vi "Begin.vi"(11 "Image Size":T1=enum."160x120") -> (0 "error out":errorcluster)   [LabVIEW 2012]
doc: "Called before other user functions, this VI is expected to open initial I/O refnums, load in file data, and do all program initialization. Notice that the <B>error out</B> terminal is simply used for data flow. Wiring it to other structures or subVIs ensures that this VI runs first."
uses:
  <vilib>/Rock Robotics/WPI/Camera/WPI_CameraImageSize.ctl
  <vilib>/Rock Robotics/WPI/Camera/WPI_CameraWhite Balance Values.ctl
  <vilib>/Rock Robotics/WPI/Camera/WPI_CameraExposure Values.ctl
  <vilib>/Rock Robotics/WPI/Camera/WPI_CameraFrameRate.ctl
  <vilib>/Rock Robotics/WPI/Joystick/WPI_JoystickDeviceEnum.ctl
  <vilib>/Rock Robotics/SystemInterfaces/DIO/FPGA_DIOPWMChannel.ctl
  <vilib>/Rock Robotics/SystemInterfaces/Typedef/FPGA_TypedefDigitalModule.ctl
  <vilib>/Rock Robotics/SystemInterfaces/DIO/FPGA_DIORelayChannel.ctl
  <vilib>/Rock Robotics/WPI/Relay/WPI_RelayDirection.ctl
  <vilib>/Rock Robotics/SystemInterfaces/AI/FPGA_AIGyroChannel.ctl
  <vilib>/Rock Robotics/SystemInterfaces/Typedef/FPGA_TypedefAnalogModuleForGyro.ctl
  <vilib>/Rock Robotics/WPI/AnalogChannel/WPI_AnalogChannelDevRef.ctl
  <vilib>/Rock Robotics/SystemInterfaces/Typedef/FPGA_TypedefAnalogModule.ctl
  <vilib>/Rock Robotics/SystemInterfaces/AI/FPGA_AIChannel.ctl
  <vilib>/Rock Robotics/SystemInterfaces/CounterEncoderSourceConvertion/FPGA_CounterEncoderSourceConvertionLVSourceType.ctl
  <vilib>/Rock Robotics/SystemInterfaces/DIO/FPGA_DIODigitalSourceChannel.ctl
  <vilib>/Rock Robotics/SystemInterfaces/AnalogTrigger/FPGA_AnalogTriggerIndex.ctl
  <vilib>/Rock Robotics/SystemInterfaces/AnalogTrigger/FPGA_AnalogTriggerOutType.ctl
  <vilib>/Rock Robotics/SystemInterfaces/DIO/FPGA_DIOChannel.ctl
  <vilib>/Rock Robotics/WPI/MotorControl/WPI_MotorControlOpen Jaguar.vi
  <vilib>/Rock Robotics/WPI/RobotDrive/WPI_RobotDriveOpen2MotorWithJaguar.vi
  <vilib>/Rock Robotics/WPI/MotorControl/WPI_MotorControlOpen Victor.vi
  <vilib>/Rock Robotics/WPI/Counter/WPI_CounterOpen UpDown Mode.vi
  <vilib>/Rock Robotics/WPI/Counter/WPI_CounterDigitalInputToDigitalSource.vi
  <vilib>/Rock Robotics/WPI/RobotDrive/WPI_RobotDriveOpen4MotorWithJaguar.vi
panel:
  out "error out 2":errorcluster
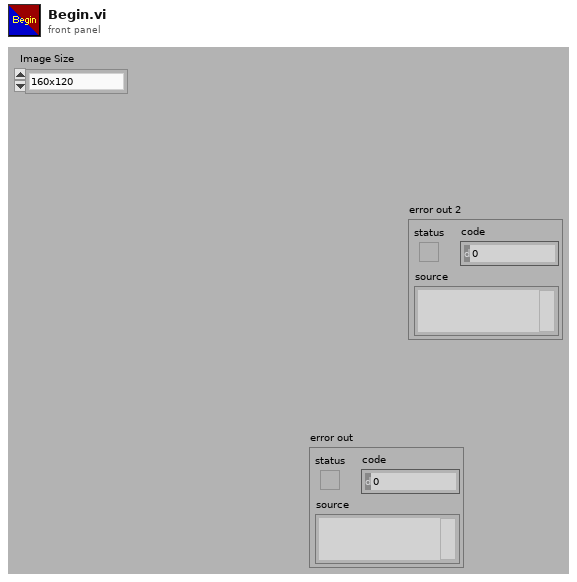
[diagram p1: front panel]
types:
  T1 = typedef "WPI_CameraImageSize.ctl" = enum16{"640x480", "320x240", "160x120"}
  T2 = typedef "FPGA_DIOPWMChannel.ctl" = enum8{"PWM 1", "PWM 2", "PWM 3", "PWM 4", "PWM 5", "PWM 6", "PWM 7", "PWM 8", "PWM 9", "PWM 10", "Invalid"}
  T3 = typedef "FPGA_TypedefDigitalModule.ctl" = enum16{"Digital Module 1", "Digital Module 2"}
  T4 = typedef "WPI_RelayDirection.ctl" = enum16{"Both directions", "Forward only", "Reverse only"}
  T5 = typedef "FPGA_DIORelayChannel.ctl" = enum8{"Relay 1", "Relay 2", "Relay 3", "Relay 4", "Relay 5", "Relay 6", "Relay 7", "Relay 8", "Invalid"}
  T6 = typedef "WPI_JoystickDeviceEnum.ctl" = enum16{"USB 1", "USB 2", "USB 3", "USB 4", "Kinect 1", "Kinect 2"}
  T7 = typedef "WPI_CameraFrameRate.ctl" = u32
  T8 = typedef "WPI_CameraExposure Values.ctl" = enum16{"Auto", "Flicker-free 50 Hz", "Flicker-free 60 Hz", "Hold current"}
  T9 = typedef "WPI_CameraWhite Balance Values.ctl" = enum16{"Auto", "Fixed indoor", "Fixed outdoor 1", "Fixed outdoor 2", "Fixed fluorescent 1", "Fixed fluorescent 2", "Hold current"}
  T10 = typedef "WPI_ServoDeviceRef.ctl" = cluster{"DeviceStatus":errorcluster, "Digital Module":T3, "PWM Channel":T2, "DeadBand":T11}
  T11 = typedef "WPI_PWMDeadband.ctl" = cluster{"Name":string, "maxPositivePwm":i32, "minPositivePwm":i32, "centerPwm":i32, "maxNegativePwm":i32, "minNegativePwm":i32, "angularRange":u16}
  T12 = typedef "WPI_MotorControlDeviceRef.ctl" = cluster{"DeviceStatus":errorcluster, "Type":enum16{"PWM", "CAN"}, "PWM":cluster{"Digital Module":T3, "PWM Channel":T2, "DeadBand":T11}, "CAN":cluster{"Device Number":u8, "Control Mode":T13, "Semaphore":T14, "Max Vout":dbl}, "Invert":bool, "TransformRef":T15, "InvTransformRef":T15}
  T13 = typedef "WPI_CANJaguar_ControlMode.ctl" = enum8{"Percent VBus", "Current", "Speed", "Position", "Voltage"}
  T14 = typedef "Semaphore RefNum" = refnum<k1>
  T15 = typedef "WPI_PWMTransform_ConPane.ctl" = refnum<vi>
  T16 = enum16{"Rising Edge", "Falling Edge", "Raising & Falling Edge", "Disabled"}
  T17 = typedef "FPGA_CounterEncoderSourceConvertionLVSourceType.ctl" = cluster{"DevStatus":errorcluster, "AnalogTriggerMode?":bool, "DigitalMode":cluster{"Digital Module":T3, "DIO Channel":T18}, "AnalogTriggerMode":cluster{"AnalogTriggerIndex":T19, "OutputType":T20}}
  T18 = typedef "FPGA_DIODigitalSourceChannel.ctl" = enum8{"DIO 1", "DIO 2", "DIO 3", "DIO 4", "DIO 5", "DIO 6", "DIO 7", "DIO 8", "DIO 9", "DIO 10", "DIO 11", "DIO 12", "DIO 13", "DIO 14", "Disabled"}
  T19 = typedef "FPGA_AnalogTriggerIndex.ctl" = enum8{"Trig 0", "Trig 1", "Trig 2", "Trig 3", "Trig 4", "Trig 5", "Trig 6", "Trig 7", "Invalid"}
  T20 = typedef "FPGA_AnalogTriggerOutType.ctl" = enum16{"InWindow", "TriggerState", "Rising", "Falling"}
  T21 = typedef "WPI_AnalogChannelDevRef.ctl" = cluster{"DevStatus":errorcluster, "Analog Module":T22, "Analog Channel":T23}
  T22 = typedef "FPGA_TypedefAnalogModule.ctl" = enum16{"Analog Module 1", "Analog Module 2"}
  T23 = typedef "FPGA_AIChannel.ctl" = enum8{"AI 1", "AI 2", "AI 3", "AI 4", "AI 5", "AI 6", "AI 7", "AI 8", "Invalid"}
  T24 = typedef "FPGA_AnalogTriggerDevRef.ctl" = cluster{"DevStatus":errorcluster, "AnalogTriggerIndex":T19}
  T25 = typedef "WPI_CounterDevRef.ctl" = cluster{"DevStatus":errorcluster, "CntIndex":T26}
  T26 = typedef "FPGA_CounterCtrSystemIndex.ctl" = enum8{"Ctr 0", "Ctr 1", "Ctr 2", "Ctr 3", "Ctr 4", "Ctr 5", "Ctr 6", "Ctr 7", "Invalid"}
  T27 = typedef "WPI_RobotDriveDevRef.ctl" = cluster{"DevStatus":errorcluster, "Motors[]":T12[], "Square Inputs":bool, "Max Output":dbl, "Isochronous":bool}
  T28 = typedef "FPGA_DIOChannel.ctl" = enum8{"DIO 1", "DIO 2", "DIO 3", "DIO 4", "DIO 5", "DIO 6", "DIO 7", "DIO 8", "DIO 9", "DIO 10", "DIO 11", "DIO 12", "DIO 13", "DIO 14", "Invalid"}
  T29 = typedef "WPI_DigitalInputDevRef.ctl" = cluster{"DevStatus":errorcluster, "DIO Channel":T28, "Digital Module":T3}
  T30 = typedef "WPI_CameraDevRef.ctl" = cluster{"Camera Address":string, "CameraStatus":errorcluster, "Acquire Image Notifier":refnum<notifier>}
  T31 = typedef "WPI_JoystickDevRef.ctl" = cluster{"Device":T6}
  T32 = typedef "WPI_RelayDevRef.ctl" = cluster{"DevStatus":errorcluster, "Relay Channel":T5, "Digital Module":T3, "Relay Direction":T4}
  T33 = typedef "FPGA_AIGyroChannel.ctl" = enum8{"AI 1", "AI 2", "Invalid"}
  T34 = typedef "FPGA_TypedefAnalogModuleForGyro.ctl" = enum16{"Analog Module 1"}
  T35 = typedef "WPI_GyroDevRef.ctl" = cluster{"DevStatus":errorcluster, "Analog Module":T22, "Analog Channel":T23, "Offset":dbl, "Gain (VoltsPerDegree/Second)":dbl}
  T36 = typedef "WPI_EncoderDevRef.ctl" = cluster{"DevStatus":errorcluster, "EncoderIndex":T37, "CounterIndex":T26, "DistancePerCount":dbl, "Decoding Type":T38}
  T37 = typedef "FPGA_EncoderIdx.ctl" = enum8{"Enc 0", "Enc 1", "Enc 2", "Enc 3", "Invalid"}
  T38 = typedef "WPI_EncoderType.ctl" = enum16{"1x", "2x", "4x"}
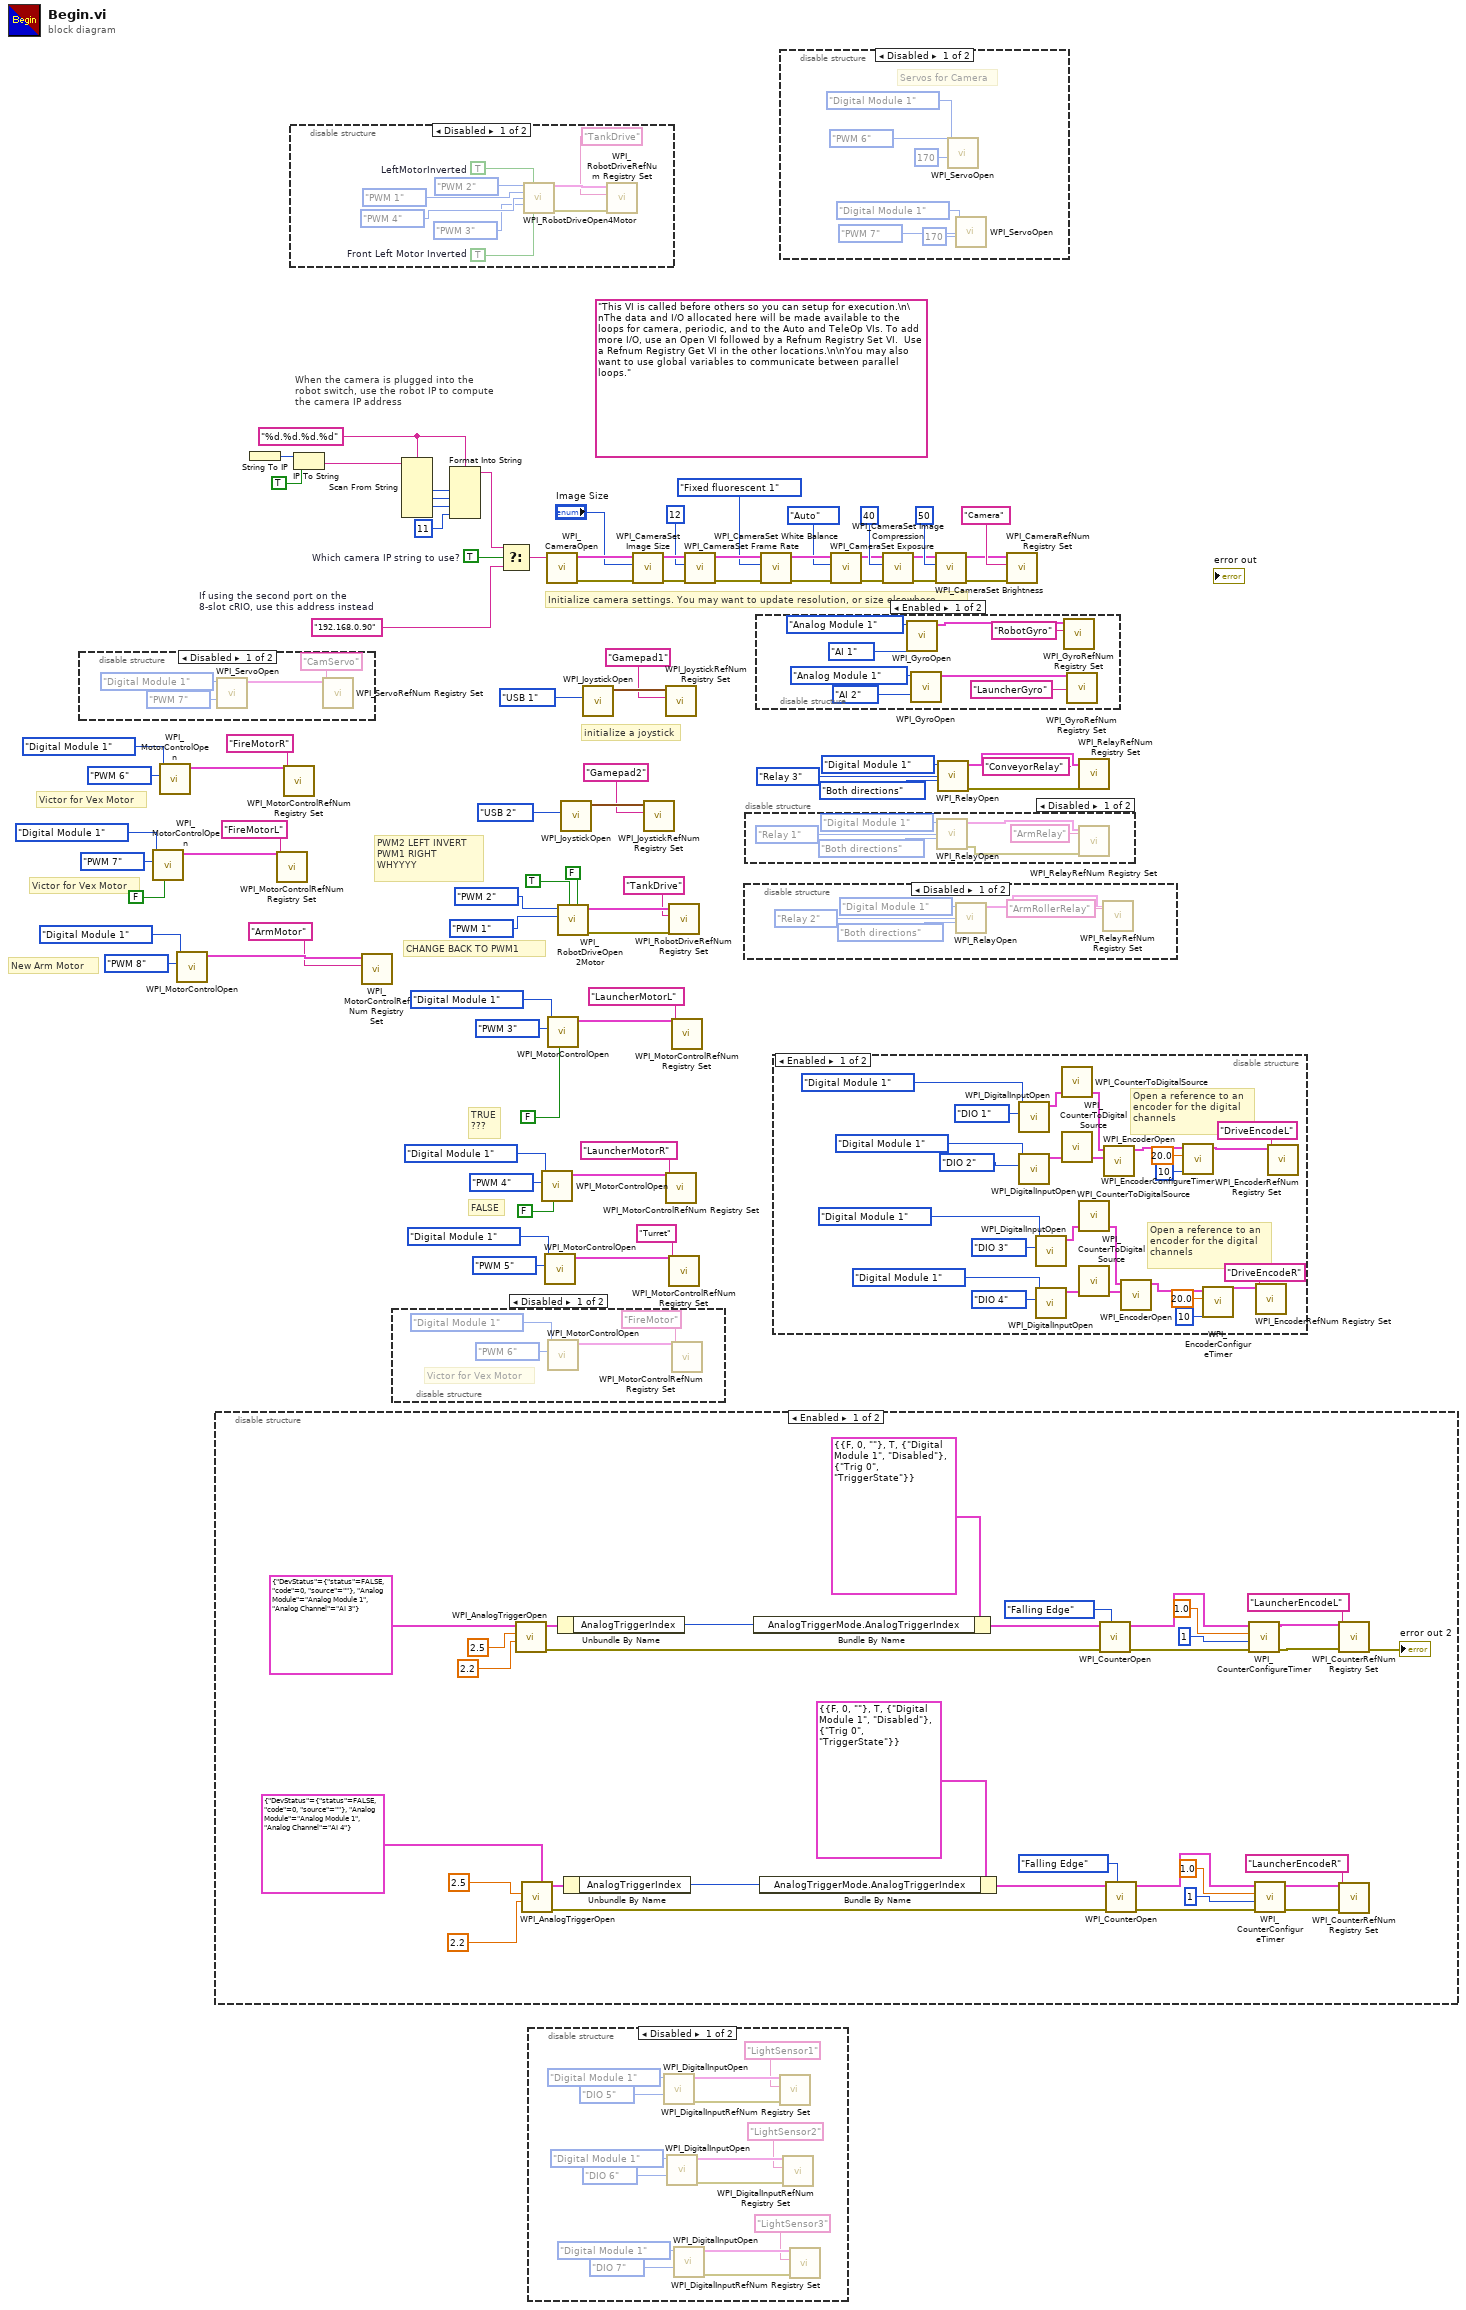
[diagram p0: block diagram]
diagram:
  w47 = TRUE  # Which camera IP string to use?
  w51 = "%d.%d.%d.%d" ("format string")
  (unwired) "This VI is called before others so you can setup for execution.\n\nThe data and I/O allocated here will be made available to the loops for camera, periodic, and to the Auto and TeleOp VIs. To add more I/O, use an Open VI followed by a Refnum Registry Set VI.  Use a Refnum Registry Get VI in the other locations.\n\nYou may also want to use global variables to communicate between parallel loops."
  w48 = "192.168.0.90"  # If using the second port on the 8-slot cRIO, use this address instead
  # "New Arm Motor"
  # "Victor for Vex Motor"
  # "Victor for Vex Motor"
  # "FALSE"
  # "TRUE\n???"
  # "PWM2 LEFT INVERT\nPWM1 RIGHT\nWHYYYY"
  # "CHANGE BACK TO PWM1"
  # "initialize a joystick"
  # "When the camera is plugged into the\nrobot switch, use the robot IP to compute\nthe camera IP address"
  # "Initialize camera settings. You may want to update resolution, or size elsewhere."
  n1 = disable-structure shown="Disabled" {
    frame Disabled {
      n2 = call <vilib>:"WPI_ServoOpen.vi"("PWM Channel"=FPGA_DIOPWMChannel."PWM 7", "Digital Module (Module 1)"=FPGA_TypedefDigitalModule."Digital Module 1") -> ("ServoDeviceRef"=w83:T10)  [unwired: 8 in, 1 out]
      n3 = call <vilib>:"WPI_ServoRefNum Registry Set.vi"("refnum name"="CamServo", "ServoDeviceRef"=w83) -> ()  [unwired: 8 in, 2 out]
    }
    frame Enabled {
    }
  }
  n4 = call-poly <vilib>:"WPI_MotorControlOpen.vi"("Invert"=FALSE, "PWM Channel"=FPGA_DIOPWMChannel."PWM 7", "Digital Module (Module 1)"=FPGA_TypedefDigitalModule."Digital Module 1") -> ("MotorControlDeviceRef"=w7:T12)  [unwired: 7 in, 1 out]
  n5 = call-poly <vilib>:"WPI_MotorControlOpen.vi"("PWM Channel"=FPGA_DIOPWMChannel."PWM 6", "Digital Module (Module 1)"=FPGA_TypedefDigitalModule."Digital Module 1") -> ("MotorControlDeviceRef"=w11:T12)  [unwired: 8 in, 1 out]
  n6 = call-poly <vilib>:"WPI_MotorControlOpen.vi"("PWM Channel"=FPGA_DIOPWMChannel."PWM 8", "Digital Module (Module 1)"=FPGA_TypedefDigitalModule."Digital Module 1") -> ("MotorControlDeviceRef"=w2:T12)  [unwired: 8 in, 1 out]
  n7 = disable-structure shown="Enabled" {
    frame Enabled {
      n8 = call <vilib>:"WPI_AnalogTriggerOpen.vi"("LowerLimit (v)"=2.2, "UpperLimit (v)"=2.5, "AnalogTriggerSource"=T21 {"DevStatus"={"status"=FALSE, "code"=0, "source"=""}, "Analog Module"=enum."Analog Module 1", "Analog Channel"=enum."AI 3"}) -> ("error out"=w115:errorcluster, "AnalogTriggerDevRef"=w108:T24)  [unwired: 7 in]
      n9 = call <vilib>:"WPI_AnalogTriggerOpen.vi"("LowerLimit (v)"=2.2 ("LowerLimit (v) 2"), "UpperLimit (v)"=2.5 ("UpperLimit (v) 2"), "AnalogTriggerSource"=T21 {"DevStatus"={"status"=FALSE, "code"=0, "source"=""}, "Analog Module"=enum."Analog Module 1", "Analog Channel"=enum."AI 4"} ("AnalogTriggerSource 2")) -> ("error out"=w102:errorcluster, "AnalogTriggerDevRef"=w95:T24)  [unwired: 7 in]
      n10 = Unbundle By Name(w108) -> ("AnalogTriggerIndex"=w107:T19)
      n11 = Unbundle By Name(w95) -> ("AnalogTriggerIndex"=w94:T19)
      n12 = Bundle By Name(cluster=T17 {"DevStatus"={"status"=FALSE, "code"=0, "source"=""}, "AnalogTriggerMode?"=TRUE, "DigitalMode"={"Digital Module"=enum."Digital Module 1", "DIO Channel"=enum."Disabled"}, "AnalogTriggerMode"={"AnalogTriggerIndex"=enum."Trig 0", "OutputType"=enum."TriggerState"}} ("Source"), "AnalogTriggerMode.AnalogTriggerIndex"=w107) -> (w105:T17)
      n13 = Bundle By Name(cluster=T17 {"DevStatus"={"status"=FALSE, "code"=0, "source"=""}, "AnalogTriggerMode?"=TRUE, "DigitalMode"={"Digital Module"=enum."Digital Module 1", "DIO Channel"=enum."Disabled"}, "AnalogTriggerMode"={"AnalogTriggerIndex"=enum."Trig 0", "OutputType"=enum."TriggerState"}} ("Source 2"), "AnalogTriggerMode.AnalogTriggerIndex"=w94) -> (w92:T17)
      n14 = call-poly <vilib>:"WPI_CounterOpen.vi"("UpEdge"=T16."Falling Edge" ("UpEdge 1"), "error in (no error)"=w115, "Up Source"=w105) -> ("error out"=w111:errorcluster, "CounterDevRef"=w112:T25)  [unwired: 7 in]
      n15 = call-poly <vilib>:"WPI_CounterOpen.vi"("UpEdge"=T16."Falling Edge" ("UpEdge 2"), "error in (no error)"=w102, "Up Source"=w92) -> ("error out"=w98:errorcluster, "CounterDevRef"=w99:T25)  [unwired: 7 in]
      n16 = call <vilib>:"WPI_CounterConfigureTimer.vi"("error in (no error)"=w111, "Number Samples to Average"=u8 1, "MaxPeriod (sec)"=1.0, "CounterDevRef in"=w112) -> ("error out"=w85:errorcluster, "CounterDevRef out"=w86:T25)  [unwired: 6 in]
      n17 = call <vilib>:"WPI_CounterConfigureTimer.vi"("error in (no error)"=w98, "Number Samples to Average"=u8 1, "MaxPeriod (sec)"=1.0, "CounterDevRef in"=w99) -> ("error out"=w89:errorcluster, "CounterDevRef out"=w90:T25)  [unwired: 6 in]
      n18 = call <vilib>:"WPI_CounterRefNum Registry Set.vi"("error in (no error)"=w85, "refnum name"="LauncherEncodeL", "CounterDevRef"=w86) -> ("error out"=→"error out 2":errorcluster)  [unwired: 7 in, 1 out]
      n19 = call <vilib>:"WPI_CounterRefNum Registry Set.vi"("error in (no error)"=w89, "refnum name"="LauncherEncodeR", "CounterDevRef"=w90) -> ()  [unwired: 7 in, 2 out]
    }
    frame Disabled {
    }
  }
  n20 = String To IP() -> (0:w58:u32)  [unwired: 1 in]
  n21 = call <vilib>:"WPI_MotorControlRefNum Registry Set.vi"("refnum name"="FireMotorL", "MotorControlDevRef"=w7) -> ()  [unwired: 8 in, 2 out]
  n22 = call <vilib>:"WPI_MotorControlRefNum Registry Set.vi"("refnum name"="FireMotorR", "MotorControlDevRef"=w11) -> ()  [unwired: 8 in, 2 out]
  n23 = disable-structure shown="Disabled" {
    frame Disabled {
      w119 = TRUE  # Front Left Motor Inverted
      w125 = TRUE  # LeftMotorInverted
      n24 = call-poly <vilib>:"WPI_RobotDriveOpen4Motor.vi"("Rear Left Motor"=FPGA_DIOPWMChannel."PWM 2" ("Left"), "Rear Left Motor Inverted"=w125, "Rear Right Motor"=FPGA_DIOPWMChannel."PWM 1" ("Right Motor"), "Front Left Motor"=FPGA_DIOPWMChannel."PWM 4", "Front Right Motor"=FPGA_DIOPWMChannel."PWM 3", "Front Left Motor Inverted"=w119) -> ("RobotDriveDevRef"=w124:T27, "error out"=w122:errorcluster)  [unwired: 8 in]
      n25 = call <vilib>:"WPI_RobotDriveRefNum Registry Set.vi"("error in (no error)"=w122, "refnum name"="TankDrive", "RobotDriveDevRef"=w124) -> ()  [unwired: 9 out]
    }
    frame Enabled {
    }
  }
  n26 = IP To String(1:TRUE ("dot notation? (F)"), 2:w58) -> (0:w56:string)
  n27 = call <vilib>:"WPI_MotorControlRefNum Registry Set.vi"("refnum name"="ArmMotor", "MotorControlDevRef"=w2) -> ()  [unwired: 8 in, 2 out]
  n28 = disable-structure shown="Disabled" {
    frame Disabled {
      # "Victor for Vex Motor"
      n29 = call-poly <vilib>:"WPI_MotorControlOpen.vi"("PWM Channel"=FPGA_DIOPWMChannel."PWM 6", "Digital Module (Module 1)"=FPGA_TypedefDigitalModule."Digital Module 1") -> ("MotorControlDeviceRef"=w127:T12)  [unwired: 8 in, 1 out]
      n30 = call <vilib>:"WPI_MotorControlRefNum Registry Set.vi"("refnum name"="FireMotor", "MotorControlDevRef"=w127) -> ()  [unwired: 8 in, 2 out]
    }
    frame Enabled {
    }
  }
  n31 = Scan From String(format string=w51, input string=w56) -> (output 1=w55:i32, output 2=w54:i32, output 3=w53:i32)  [unwired: 7 in, 3 out]
  n32 = Format Into String(format string=w51, w55, w54, w53, 11 ("Compression")) -> (resulting string=w49:string)  [unwired: 2 in, 1 out]
  n33 = Select(t=w49, s=w47, f=w48) -> (s? t:f=w50:string)
  n34 = disable-structure shown="Disabled" {
    frame Disabled {
      n35 = call <vilib>:"WPI_DigitalInputOpen.vi"("DIO Channel"=FPGA_DIOChannel."DIO 5", "Digital Module (Module 1)"=FPGA_TypedefDigitalModule."Digital Module 1") -> ("error out"=w141:errorcluster, "DigitalInputDevRef"=w142:T29)  [unwired: 8 in]
      n36 = call <vilib>:"WPI_DigitalInputOpen.vi"("DIO Channel"=FPGA_DIOChannel."DIO 6", "Digital Module (Module 1)"=FPGA_TypedefDigitalModule."Digital Module 1") -> ("error out"=w136:errorcluster, "DigitalInputDevRef"=w137:T29)  [unwired: 8 in]
      n37 = call <vilib>:"WPI_DigitalInputOpen.vi"("DIO Channel"=FPGA_DIOChannel."DIO 7", "Digital Module (Module 1)"=FPGA_TypedefDigitalModule."Digital Module 1") -> ("error out"=w131:errorcluster, "DigitalInputDevRef"=w132:T29)  [unwired: 8 in]
      n38 = call <vilib>:"WPI_DigitalInputRefNum Registry Set.vi"("error in (no error)"=w141, "refnum name"="LightSensor1", "DigitalInputDevRef"=w142) -> ()  [unwired: 7 in, 2 out]
      n39 = call <vilib>:"WPI_DigitalInputRefNum Registry Set.vi"("error in (no error)"=w136, "refnum name"="LightSensor2", "DigitalInputDevRef"=w137) -> ()  [unwired: 7 in, 2 out]
      n40 = call <vilib>:"WPI_DigitalInputRefNum Registry Set.vi"("error in (no error)"=w131, "refnum name"="LightSensor3", "DigitalInputDevRef"=w132) -> ()  [unwired: 7 in, 2 out]
    }
    frame Enabled {
    }
  }
  n41 = call-poly <vilib>:"WPI_MotorControlOpen.vi"("Invert"=FALSE, "PWM Channel"=FPGA_DIOPWMChannel."PWM 4", "Digital Module (Module 1)"=FPGA_TypedefDigitalModule."Digital Module 1") -> ("MotorControlDeviceRef"=w29:T12)  [unwired: 7 in, 1 out]
  n42 = call-poly <vilib>:"WPI_MotorControlOpen.vi"("PWM Channel"=FPGA_DIOPWMChannel."PWM 5", "Digital Module (Module 1)"=FPGA_TypedefDigitalModule."Digital Module 1") -> ("MotorControlDeviceRef"=w25:T12)  [unwired: 8 in, 1 out]
  n43 = call <vilib>:"WPI_CameraOpen.vi"("Camera Address"=w50) -> ("error out"=w70:errorcluster, "CameraDevRef"=w71:T30)  [unwired: 1 in, 8 out]
  n44 = call-poly <vilib>:"WPI_MotorControlOpen.vi"("Invert"=FALSE, "PWM Channel"=FPGA_DIOPWMChannel."PWM 3", "Digital Module (Module 1)"=FPGA_TypedefDigitalModule."Digital Module 1") -> ("MotorControlDeviceRef"=w33:T12)  [unwired: 7 in, 1 out]
  n45 = call-poly <vilib>:"WPI_RobotDriveOpen2Motor.vi"("Right Motor Inverted"=FALSE, "Left Motor Inverted"=TRUE, "Right Motor"=FPGA_DIOPWMChannel."PWM 1", "Left Motor"=FPGA_DIOPWMChannel."PWM 2") -> ("error out"=w36:errorcluster, "RobotDriveDevRef"=w40:T27)  [unwired: 6 in]
  n46 = call <vilib>:"WPI_JoystickOpen.vi"("JoystickDevice"=WPI_JoystickDeviceEnum."USB 2") -> ("JoystickDevRef"=w43:T31)  [unwired: 10 out]
  n47 = call <vilib>:"WPI_JoystickOpen.vi"("JoystickDevice"=WPI_JoystickDeviceEnum."USB 1") -> ("JoystickDevRef"=w46:T31)  [unwired: 10 out]
  n48 = call <vilib>:"WPI_CameraSet Image Size.vi"("error in (no error)"=w70, "Image Size"="Image Size", "CameraDevRef"=w71) -> ("error out"=w69:errorcluster, "CameraDevRef Out"=w72:T30)  [unwired: 7 out]
  n49 = call <vilib>:"WPI_JoystickRefNum Registry Set.vi"("refnum name"="Gamepad2", "JoystickDevRef"=w43) -> ()  [unwired: 1 in, 9 out]
  n50 = call <vilib>:"WPI_JoystickRefNum Registry Set.vi"("refnum name"="Gamepad1", "JoystickDevRef"=w46) -> ()  [unwired: 1 in, 9 out]
  n51 = call <vilib>:"WPI_MotorControlRefNum Registry Set.vi"("refnum name"="LauncherMotorR", "MotorControlDevRef"=w29) -> ()  [unwired: 8 in, 2 out]
  n52 = call <vilib>:"WPI_RobotDriveRefNum Registry Set.vi"("error in (no error)"=w36, "refnum name"="TankDrive", "RobotDriveDevRef"=w40) -> ()  [unwired: 7 in, 2 out]
  n53 = call <vilib>:"WPI_MotorControlRefNum Registry Set.vi"("refnum name"="Turret", "MotorControlDevRef"=w25) -> ()  [unwired: 8 in, 2 out]
  n54 = call <vilib>:"WPI_MotorControlRefNum Registry Set.vi"("refnum name"="LauncherMotorL", "MotorControlDevRef"=w33) -> ()  [unwired: 8 in, 2 out]
  n55 = call <vilib>:"WPI_CameraSet Frame Rate.vi"("error in (no error)"=w69, "Frame Rate (fps)"=T7 12, "CameraDevRef"=w72) -> ("error out"=w68:errorcluster, "CameraDevRef Out"=w74:T30)  [unwired: 7 out]
  n56 = disable-structure shown="Disabled" {
    frame Disabled {
      n57 = call <vilib>:"WPI_RelayOpen.vi"("Relay Direction"=WPI_RelayDirection."Both directions", "Relay Channel"=FPGA_DIORelayChannel."Relay 2", "Digital Module (Module 1)"=FPGA_TypedefDigitalModule."Digital Module 1") -> ("RelayDevRef"=w145:T32)  [unwired: 7 in, 1 out]
      n58 = call <vilib>:"WPI_RelayRefNum Registry Set.vi"("refnum name"="ArmRollerRelay", "RelayDevRef"=w145) -> ()  [unwired: 8 in, 2 out]
    }
    frame Enabled {
    }
  }
  n59 = disable-structure shown="Disabled" {
    frame Disabled {
      n60 = call <vilib>:"WPI_RelayOpen.vi"("Relay Direction"=WPI_RelayDirection."Both directions", "Relay Channel"=FPGA_DIORelayChannel."Relay 1", "Digital Module (Module 1)"=FPGA_TypedefDigitalModule."Digital Module 1") -> ("error out"=w150:errorcluster, "RelayDevRef"=w151:T32)  [unwired: 7 in]
      n61 = call <vilib>:"WPI_RelayRefNum Registry Set.vi"("error in (no error)"=w150, "refnum name"="ArmRelay", "RelayDevRef"=w151) -> ()  [unwired: 7 in, 2 out]
    }
    frame Enabled {
    }
  }
  n62 = disable-structure shown="Enabled" {
    frame Enabled {
      n63 = call <vilib>:"WPI_GyroOpen.vi"("Analog Channel"=FPGA_AIGyroChannel."AI 1", "Analog Module (Module 1)"=FPGA_TypedefAnalogModuleForGyro."Analog Module 1") -> ("GyroDevRef"=w159:T35)  [unwired: 7 in, 2 out]
      n64 = call <vilib>:"WPI_GyroOpen.vi"("Analog Channel"=FPGA_AIGyroChannel."AI 2", "Analog Module (Module 1)"=FPGA_TypedefAnalogModuleForGyro."Analog Module 1") -> ("GyroDevRef"=w158:T35)  [unwired: 7 in, 2 out]
      n65 = call <vilib>:"WPI_GyroRefNum Registry Set.vi"("refnum name"="RobotGyro", "GyroDevRef"=w159) -> ()  [unwired: 8 in, 2 out]
      n66 = call <vilib>:"WPI_GyroRefNum Registry Set.vi"("refnum name"="LauncherGyro", "GyroDevRef"=w158) -> ()  [unwired: 8 in, 2 out]
    }
    frame Disabled {
    }
  }
  n67 = call <vilib>:"WPI_CameraSet White Balance.vi"("error in (no error)"=w68, "White Balance"=WPI_CameraWhite_Balance_Values."Fixed fluorescent 1", "CameraDevRef"=w74) -> ("error out"=w67:errorcluster, "CameraDevRef Out"=w73:T30)  [unwired: 7 out]
  n68 = disable-structure shown="Enabled" {
    frame Enabled {
      # "Open a reference to an\nencoder for the digital \nchannels"
      # "Open a reference to an\nencoder for the digital \nchannels"
      n69 = call <vilib>:"WPI_DigitalInputOpen.vi"("DIO Channel"=FPGA_DIOChannel."DIO 1", "Digital Module (Module 1)"=FPGA_TypedefDigitalModule."Digital Module 1") -> ("DigitalInputDevRef"=w187:T29)  [unwired: 1 in, 8 out]
      n70 = call <vilib>:"WPI_DigitalInputOpen.vi"("DIO Channel"=FPGA_DIOChannel."DIO 2", "Digital Module (Module 1)"=FPGA_TypedefDigitalModule."Digital Module 1") -> ("DigitalInputDevRef"=w188:T29)  [unwired: 1 in, 8 out]
      n71 = call <vilib>:"WPI_DigitalInputOpen.vi"("DIO Channel"=FPGA_DIOChannel."DIO 3", "Digital Module (Module 1)"=FPGA_TypedefDigitalModule."Digital Module 1") -> ("DigitalInputDevRef"=w177:T29)  [unwired: 1 in, 8 out]
      n72 = call <vilib>:"WPI_DigitalInputOpen.vi"("DIO Channel"=FPGA_DIOChannel."DIO 4", "Digital Module (Module 1)"=FPGA_TypedefDigitalModule."Digital Module 1") -> ("DigitalInputDevRef"=w178:T29)  [unwired: 1 in, 8 out]
      n73 = call-poly <vilib>:"WPI_CounterToDigitalSource.vi"("DigitalInputDevRef"=w187) -> ("Digital Source"=w186:T17)  [unwired: 6 out]
      n74 = call-poly <vilib>:"WPI_CounterToDigitalSource.vi"("DigitalInputDevRef"=w188) -> ("Digital Source"=w189:T17)  [unwired: 6 out]
      n75 = call-poly <vilib>:"WPI_CounterToDigitalSource.vi"("DigitalInputDevRef"=w177) -> ("Digital Source"=w176:T17)  [unwired: 6 out]
      n76 = call-poly <vilib>:"WPI_CounterToDigitalSource.vi"("DigitalInputDevRef"=w178) -> ("Digital Source"=w179:T17)  [unwired: 6 out]
      n77 = call <vilib>:"WPI_EncoderOpen.vi"("BSource"=w189, "ASource"=w186) -> ("EncoderDevRef"=w183:T36)  [unwired: 6 in, 3 out]
      n78 = call <vilib>:"WPI_EncoderOpen.vi"("BSource"=w179, "ASource"=w176) -> ("EncoderDevRef"=w175:T36)  [unwired: 6 in, 3 out]
      n79 = call <vilib>:"WPI_EncoderConfigureTimer.vi"("Number Samples to Average"=u8 10, "Minimum Rate"=20.0, "EncoderDevRef"=w183) -> ("EncoderDevRef"=w180:T36)  [unwired: 1 in, 7 out]
      n80 = call <vilib>:"WPI_EncoderConfigureTimer.vi"("Number Samples to Average"=u8 10, "Minimum Rate"=20.0, "EncoderDevRef"=w175) -> ("EncoderDevRef"=w172:T36)  [unwired: 1 in, 7 out]
      n81 = call <vilib>:"WPI_EncoderRefNum Registry Set.vi"("refnum name"="DriveEncodeR", "EncoderDevRef"=w172) -> ()  [unwired: 8 in, 2 out]
      n82 = call <vilib>:"WPI_EncoderRefNum Registry Set.vi"("refnum name"="DriveEncodeL", "EncoderDevRef"=w180) -> ()  [unwired: 8 in, 2 out]
    }
    frame Disabled {
    }
  }
  n83 = disable-structure shown="Disabled" {
    frame Disabled {
      # "Servos for Camera"
      n84 = call <vilib>:"WPI_ServoOpen.vi"("Angular Range"=u16 170, "PWM Channel"=FPGA_DIOPWMChannel."PWM 6", "Digital Module (Module 1)"=FPGA_TypedefDigitalModule."Digital Module 1") -> ()  [unwired: 7 in, 2 out]
      n85 = call <vilib>:"WPI_ServoOpen.vi"("Angular Range"=u16 170, "PWM Channel"=FPGA_DIOPWMChannel."PWM 7", "Digital Module (Module 1)"=FPGA_TypedefDigitalModule."Digital Module 1") -> ()  [unwired: 7 in, 2 out]
    }
    frame Enabled {
    }
  }
  n86 = call <vilib>:"WPI_CameraSet Exposure.vi"("error in (no error)"=w67, "Exposure"=WPI_CameraExposure_Values."Auto", "CameraDevRef"=w73) -> ("error out"=w66:errorcluster, "CameraDevRef Out"=w76:T30)  [unwired: 7 out]
  n87 = call <vilib>:"WPI_CameraSet Image Compression.vi"("error in (no error)"=w66, "Compression"=40, "CameraDevRef"=w76) -> ("error out"=w65:errorcluster, "CameraDevRef Out"=w75:T30)  [unwired: 7 out]
  n88 = call <vilib>:"WPI_CameraSet Brightness.vi"("error in (no error)"=w65, "Brightness"=50, "CameraDevRef"=w75) -> ("error out"=w63:errorcluster, "CameraDevRef Out"=w64:T30)  [unwired: 7 out]
  n89 = call <vilib>:"WPI_RelayOpen.vi"("Relay Direction"=WPI_RelayDirection."Both directions", "Relay Channel"=FPGA_DIORelayChannel."Relay 3", "Digital Module (Module 1)"=FPGA_TypedefDigitalModule."Digital Module 1") -> ("error out"=w14:errorcluster, "RelayDevRef"=w21:T32)  [unwired: 7 in]
  n90 = call <vilib>:"WPI_CameraRefNum Registry Set.vi"("error in (no error)"=w63, "refnum name"="Camera", "CameraDevRef"=w64) -> ()  [unwired: 9 out]
  n91 = call <vilib>:"WPI_RelayRefNum Registry Set.vi"("error in (no error)"=w14, "refnum name"="ConveyorRelay", "RelayDevRef"=w21) -> ()  [unwired: 7 in, 2 out]
